vi "Cleanup.vi"(8 "error in (no error)":errorcluster, 11 "Start Pre-Soak in":refnum<class "Wait.lvclass">) -> (0 "error out":errorcluster, 3 "Start Pre-Soak out":refnum<class "Wait.lvclass">)   [LabVIEW 2019, in "Wait.lvclass"]
uses:
  <vilib>/gpm_packages/@cs/Car-wash/Source/Process Steps/Wait/Wait.lvclass
  <vilib>/gpm_packages/@cs/Car-wash/Source/Process Steps/Wait/Wait.lvclass/Wait.ctl
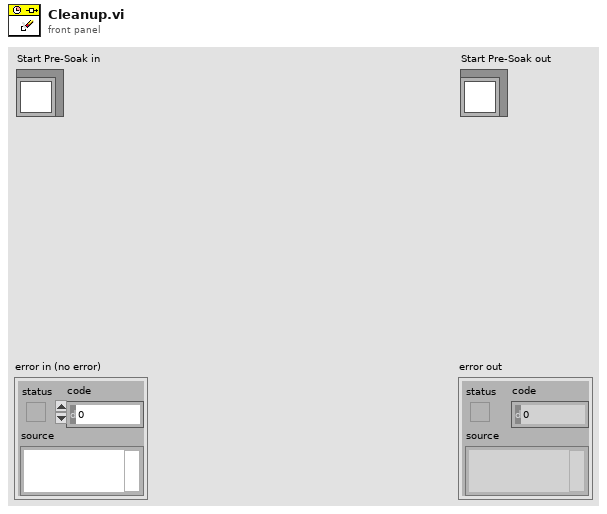
[diagram p1: front panel]
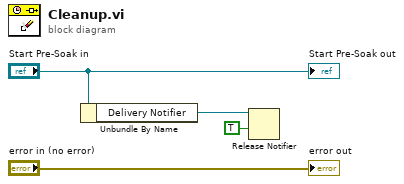
[diagram p0: block diagram]
diagram:
  n1 = Unbundle By Name("Start Pre-Soak in") -> ("Delivery Notifier"=w2:refnum<notifier>)
  n2 = Release Notifier(notifier=w2, force destroy? (F)=TRUE) -> ()  [unwired: 1 in, 3 out]
  "error out" <- "error in (no error)"
  "Start Pre-Soak out" <- "Start Pre-Soak in"
